vi "Arrange Indicators in 2D Array.vi"(8 "controls":refnum<vi>[](array[refnum]), 9 "indicators":refnum<vi>[](array[refnum]), 10 "indicators seqence":T1(array[cluster]), 11 "2-D references array":refnum<vi>[][](array[refnum])) -> (3 "2-D references array out":refnum<vi>[][](array[refnum]))   [LabVIEW 2018, in "NISAST VI Scripting.lvlib" / "VI.lvlib" / "Front Panel.lvlib"]
uses:
  Front Panel.lvlib
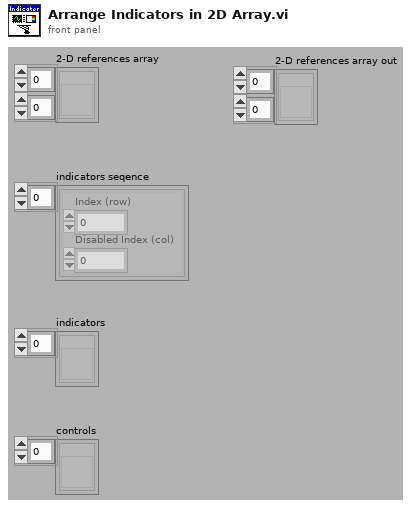
[diagram p1: front panel]
types:
  T1 = cluster{"Index (row)":i32, "Disabled Index (col)":i32}[]
  T2 = cluster{"Index (row)":i32, "Disabled Index (col)":i32}
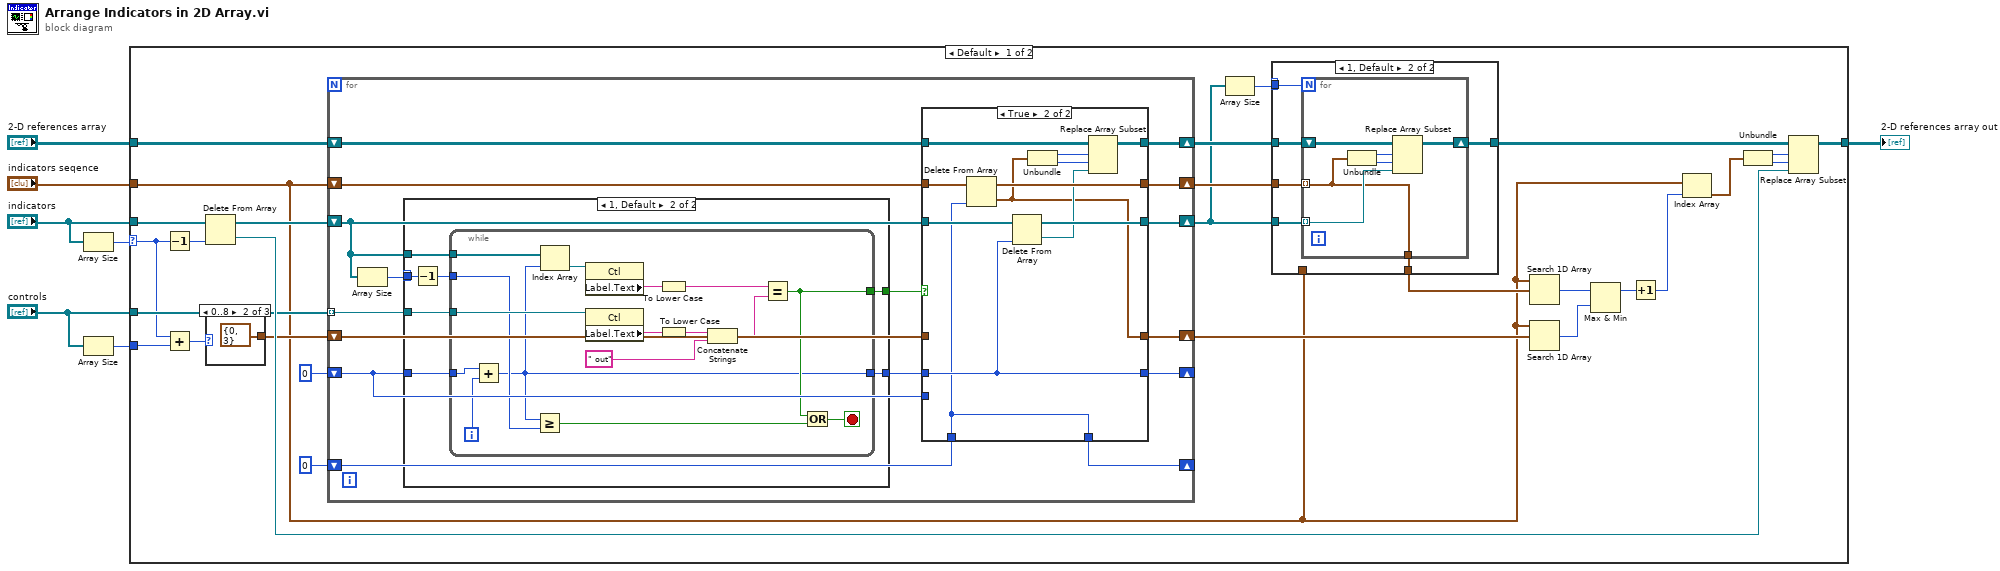
[diagram p0: block diagram]
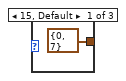
[diagram p2: hidden frame]
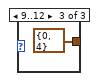
[diagram p3: hidden frame]
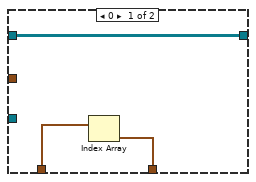
[diagram p4: hidden frame]
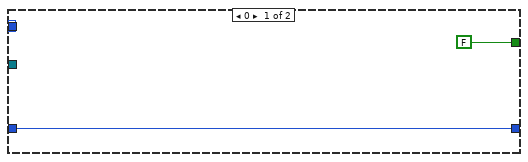
[diagram p5: hidden frame]
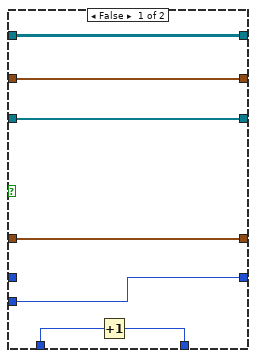
[diagram p6: hidden frame]
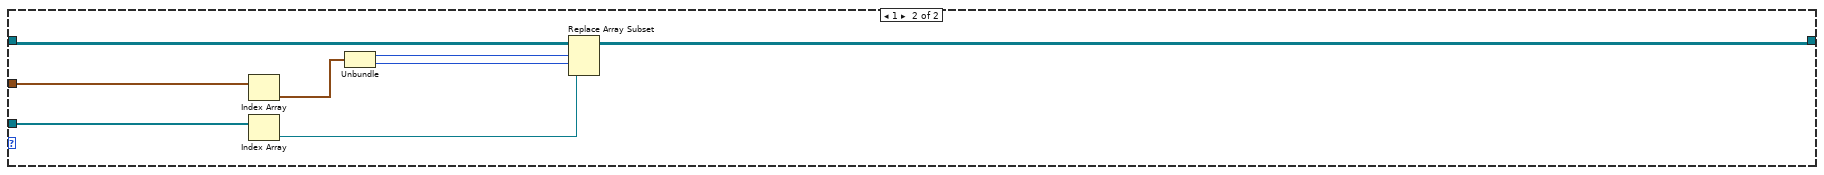
[diagram p7: hidden frame]
diagram:
  n1 = Array Size(array="indicators") -> (size(s)=w3:i32)
  n2 = Array Size(array="controls") -> (size(s)=w1:i32)
  n3 = case shown="Default" w3 {
    selector: w3 -> [w9 _]
    tunnel: "indicators seqence" -> [w12 w121]
    tunnel: [w30 w114] -> w6
    tunnel: "controls" -> [w18 _]
    tunnel: "2-D references array" -> [w17 w115]
    tunnel: "indicators" -> [w16 w117]
    tunnel: w1 -> [w10 _]
    frame Default {
      n4 = Decrement(x=w9) -> (x-1=w15:i32)
      n5 = Add(x=w9, y=w10) -> (x+y=w8:i32)
      n6 = Delete From Array(array=w16, index=w15) -> (deleted portion=w35:refnum<vi>, array with subset deleted=w20:refnum<vi>[])  [unwired: 1 in]
      n7 = case shown="0..8" w8 {
        tunnel: [T2 {"Index (row)"=0, "Disabled Index (col)"=7} T2 {"Index (row)"=0, "Disabled Index (col)"=3} T2 {"Index (row)"=0, "Disabled Index (col)"=4}] -> w26
        frame 15, Default {
        }
        frame 0..8 {
        }
        frame 9..12 {
        }
      }
      n8 = for {
        shift-right: [w65] -> w21
        shift-left: w17 -> [w66]
        tunnel: w18 -> [w69] mode=indexing
        shift-right: [w64] -> _
        shift-left: 0 -> [w61]
        shift-right: [w63] -> w22
        shift-left: w12 -> [w67]
        shift-right: [w62] -> w14
        shift-left: w20 -> [w60]
        shift-right: [w58] -> w25
        shift-left: w26 -> [w57]
        shift-right: [w55] -> _
        shift-left: 0 -> [w56]
        n9 = Array Size(array=w60) -> (size(s)=w54:i32)
        n10 = case shown="1, Default" w54 {
          tunnel: w69 -> [_ w78]
          tunnel: [FALSE w77] -> w68
          tunnel: w61 -> [w70 w76]
          tunnel: w60 -> [_ w75]
          tunnel: [w70 w74] -> w59
          tunnel: w54 -> [_ w72]
          frame 0 {
          }
          frame 1, Default {
            n11 = Decrement(x=w72) -> (x-1=w73:i32)
            n12 = while {
              tunnel: w78 -> [w94]
              tunnel: [w82] -> w77
              tunnel: w75 -> [w86]
              tunnel: w76 -> [w85]
              tunnel: w73 -> [w80]
              tunnel: [w79] -> w74
              i -> [w84]
              stop <- w83 stop-if-true
              n13 = Add(x=w85, y=w84) -> (x+y=w79:i32)
              n14 = Greater Or Equal?(x=w79, y=w80) -> (x >= y?=w81:bool)
              n15 = Index Array(array=w86, index=w79) -> (element=w87:refnum<vi>)
              n16 = property class="Ctl"(reference=w87) -> ("Label.Text"=w93:string)  [unwired: 1 in, 2 out]
              n17 = property class="Ctl"(reference=w94) -> ("Label.Text"=w92:string)  [unwired: 1 in, 2 out]
              n18 = To Lower Case(string=w93) -> (all lower case string=w88:string)
              n19 = To Lower Case(string=w92) -> (all lower case string=w91:string)
              n20 = Concatenate Strings(w91, " out") -> (w89:string)
              n21 = Equal?(x=w88, y=w89) -> (x = y?=w82:bool)
              n22 = Or(x=w82, y=w81) -> (x .or. y?=w83:bool)
            }
          }
        }
        n23 = case shown="True" w68 {
          tunnel: w67 -> [w99 w109]
          tunnel: w66 -> [w101 w111]
          tunnel: [w101 w110] -> w65
          tunnel: w61 -> [w100 _]
          tunnel: [w100 w105] -> w64
          tunnel: w60 -> [w98 w107]
          tunnel: [w99 w108] -> w63
          tunnel: w56 -> [w96 w102]
          tunnel: [w98 w106] -> w62
          tunnel: w59 -> [_ w105]
          tunnel: [w97 w103] -> w58
          tunnel: w57 -> [w97 _]
          tunnel: [w95 w102] -> w55
          frame False {
            n24 = Increment(x=w96) -> (x+1=w95:i32)
          }
          frame True {
            n25 = Delete From Array(array=w109, index=w102) -> (deleted portion=w103:T2, array with subset deleted=w108:T1)  [unwired: 1 in]
            n26 = Delete From Array(array=w107, index=w105) -> (deleted portion=w104:refnum<vi>, array with subset deleted=w106:refnum<vi>[])  [unwired: 1 in]
            n27 = Unbundle(w103) -> ("Index (row)"=w112:i32, "Disabled Index (col)"=w113:i32)
            n28 = Replace Array Subset(array=w111, new element=w104, index (row)=w112, index (col)=w113) -> (w110:refnum<vi>[][])
          }
        }
      }
      n29 = Array Size(array=w14) -> (size(s)=w13:i32)
      n30 = case shown="1, Default" w13 {
        tunnel: [w41 w47] -> w29
        tunnel: [w40 w46] -> w23
        tunnel: w22 -> [_ w45]
        tunnel: w21 -> [w41 w44]
        tunnel: w13 -> [_ w43]
        tunnel: w14 -> [_ w42]
        tunnel: w12 -> [w39 _]
        frame 0 {
          n31 = Index Array(array=w39) -> (element=w40:T2)  [unwired: 1 in]
        }
        frame 1, Default {
          n32 = for {
            N: w43 -> [_]
            tunnel: w42 -> [w49] mode=indexing
            shift-right: [w52] -> w47
            shift-left: w44 -> [w53]
            tunnel: w45 -> [w48] mode=indexing
            tunnel: [w48] -> w46
            n33 = Unbundle(w48) -> ("Index (row)"=w51:i32, "Disabled Index (col)"=w50:i32)
            n34 = Replace Array Subset(array=w53, new element=w49, index (row)=w51, index (col)=w50) -> (w52:refnum<vi>[][])
          }
        }
      }
      n35 = Search 1D Array(1D array=w12, element=w23) -> (index of element=w24:i32)  [unwired: 1 out]
      n36 = Search 1D Array(1D array=w12, element=w25) -> (index of element=w27:i32)  [unwired: 1 in]
      n37 = Max & Min(x=w24, y=w27) -> (max(x,y)=w28:i32)  [unwired: 1 out]
      n38 = Increment(x=w28) -> (x+1=w31:i32)
      n39 = Index Array(array=w12, index=w31) -> (element=w32:T2)
      n40 = Unbundle(w32) -> ("Index (row)"=w33:i32, "Disabled Index (col)"=w34:i32)
      n41 = Replace Array Subset(array=w29, new element=w35, index (row)=w33, index (col)=w34) -> (w30:refnum<vi>[][])
    }
    frame 1 {
      n42 = Index Array(array=w121) -> (element=w120:T2)  [unwired: 1 in]
      n43 = Index Array(array=w117) -> (element=w116:refnum<vi>)  [unwired: 1 in]
      n44 = Unbundle(w120) -> ("Index (row)"=w119:i32, "Disabled Index (col)"=w118:i32)
      n45 = Replace Array Subset(array=w115, new element=w116, index (row)=w119, index (col)=w118) -> (w114:refnum<vi>[][])
    }
  }
  "2-D references array out" <- w6
